vi "StringifiedData.vi"(8 "error in (no error)":errorcluster, 11 "PathArrayMsg in":refnum<class "PathArrayMsg.lvclass">) -> (0 "error out":errorcluster, 2 "Stringified Data":string, 3 "PathArrayMsg out":refnum<class "PathArrayMsg.lvclass">)   [LabVIEW 2018, in "LapDog.Messaging.v3.NativeArrays.lvlib" / "PathArrayMsg.lvclass"]
doc: "This VI is used for the message probe. Child classes may override it and provide the message data in string format or a short string describing the data the message contains. This string will be displayed in the probe window."
uses:
  PathArrayMsg.lvclass
  PathArrayMsg.lvclass/PathArrayMsg.ctl
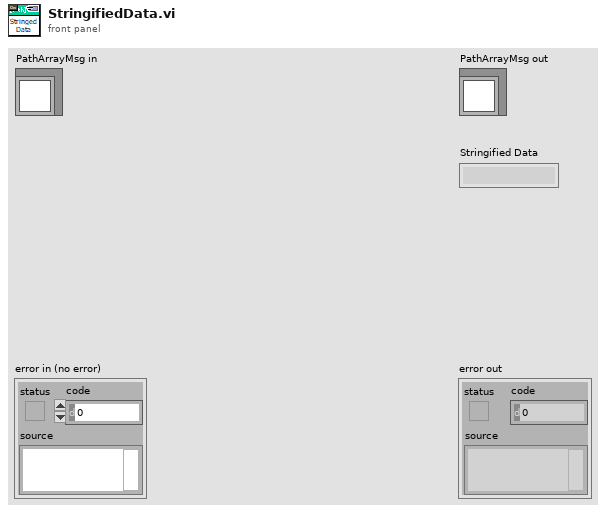
[diagram p1: front panel]
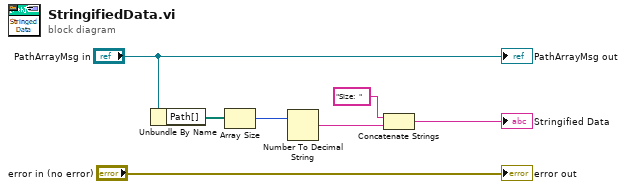
[diagram p0: block diagram]
diagram:
  n1 = Unbundle By Name("PathArrayMsg in") -> ("Path[]"=w6:path[])
  n2 = Array Size(array=w6) -> (size(s)=w5:i32)
  n3 = Number To Decimal String(number=w5) -> (decimal integer string=w3:string)  [unwired: 1 in]
  n4 = Concatenate Strings("Size:  " ("string"), w3) -> (→"Stringified Data":string)
  "error out" <- "error in (no error)"
  "PathArrayMsg out" <- "PathArrayMsg in"
